vi "Mode 3 - GUI.vi"() -> ()   [LabVIEW 2020]
uses:
  <vilib>/Platform/TimedLoop/XDataNode/timing_clust.ctl
  <vilib>/Platform/TimedLoop/XDataNode/nitl_modes.ctl
  <vilib>/Platform/TimedLoop/XDataNode/wakeup.ctl
  <vilib>/Instr/_visa.llb/VISA Configure Serial Port (Instr).vi
  <vilib>/platform/TimedLoop/XDataNode/XDataNode.xnode
  <vilib>/Platform/TimedLoop/XDataNode/XDNodeRunTimeDep.lvlib
panel:
  in  "byte count":u32=31
  in  "Slider 3 Counter":i32
  out "Blue Workpiece":bool
  out "Counter Up ?":bool
  in  "Slider 2 Counter":i32
  in  "Slider 1 Counter":i32
  out "Green Workpiece":bool
  out "Red Workpiece":bool
  in  "STOP":bool
  in  "VISA resource name":refnum<visa-resource-name>
  out "Report Data":string
  # "TRAINER ARDUINO\nMPS SORTING STATION"
  # "Mechatronics Engineering 2nd Generation\n  Vocational High School 2 Bojonegoro\n2021"
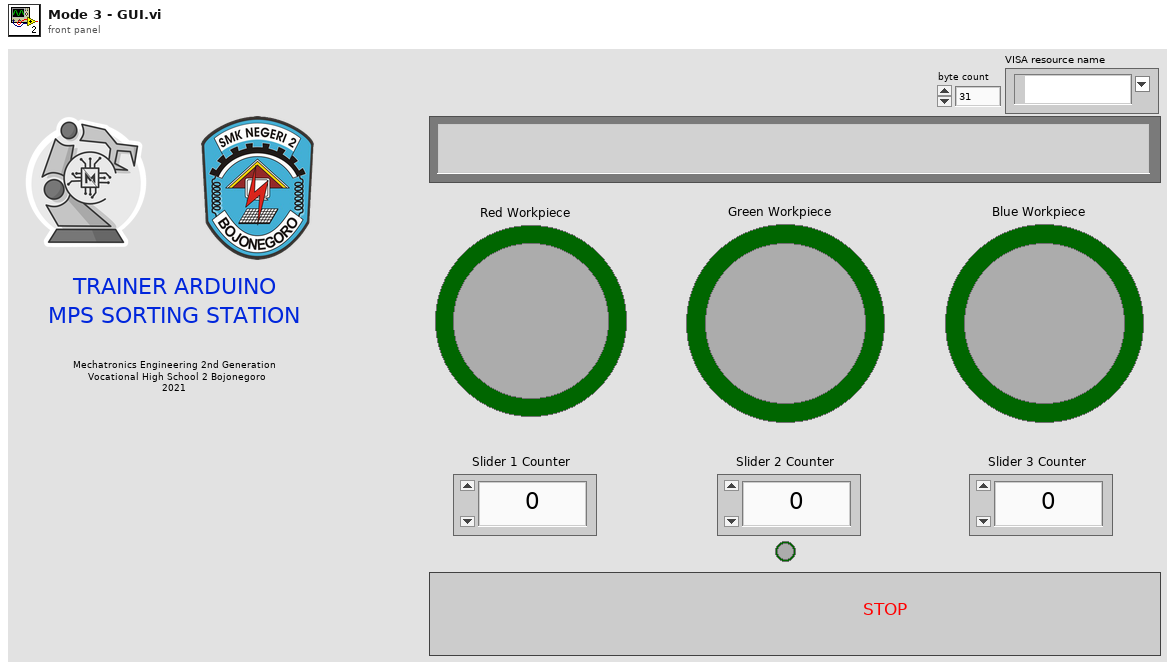
[diagram p1: front panel]
types:
  T1 = typedef "XDNodeRunTimeDep.lvlib/timing_clust.ctl" = cluster{"Expected End [f-1]":u64, "Actual End [f-1]":u64, "Finished Late? [f-1]":bool, "Expected End [i-1]":u64, "Actual End [i-1]":u64, "Finished Late? [i-1]":bool, "Expected Start [i]":u64, "Actual Start [i]":u64, "Expected Start [f]":u64, "Actual Start [f]":u64, "Source Name":string, "Structure Name":string, "Period":i64, "Deadline":i64, "Offset":i64, "Start":i64, "Priority":i32, "Timeout":i32, "Mode":T2, "Wakeup Reason":T3, "Error":errorcluster, "Source Type":string, "Secondary Source Type":string, "Global End Time":u64, "Global Start Time":u64, "Frame Duration":u64, "Iteration Duration":u64, "Assigned CPU":i32, "I/O Scan Engine Mode":u32}
  T2 = typedef "XDNodeRunTimeDep.lvlib/nitl_modes.ctl" = enum32{"No Change", "Process missed periods, maintain original phase", "Discard missed periods, maintain original phase", "Process missed periods, ignore original phase", "Discard missed periods, ignore original phase"}
  T3 = typedef "XDNodeRunTimeDep.lvlib/wakeup.ctl" = enum32{"Normal", "Aborted", "Asynchronous wakeup", "Timing source error", "Timed loop error", "Timeout"}
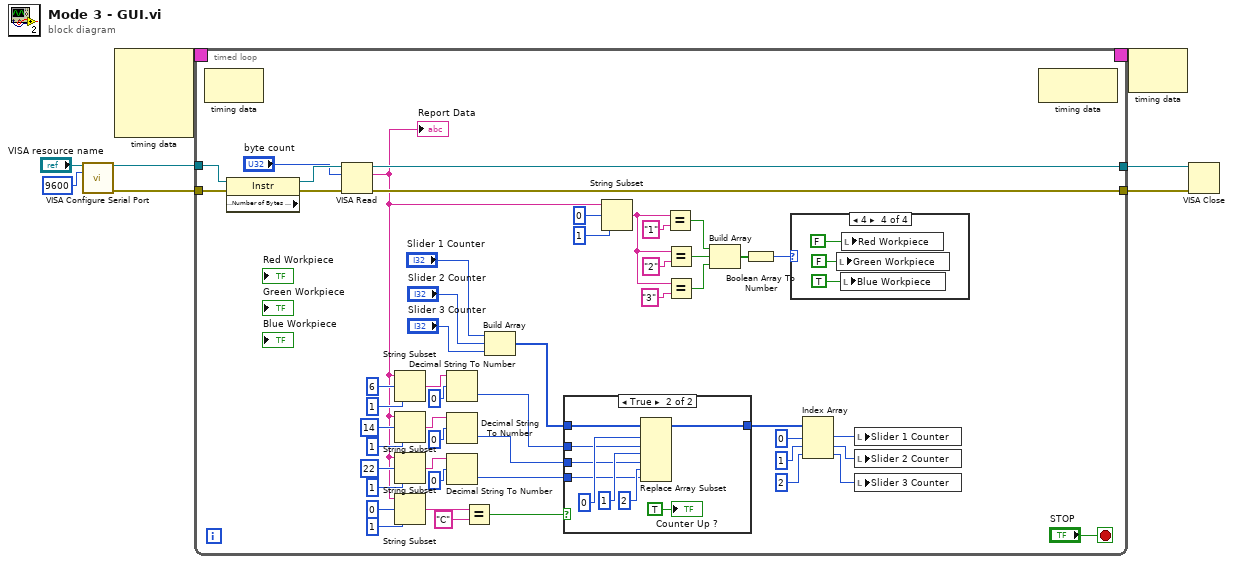
[diagram p0: block diagram]
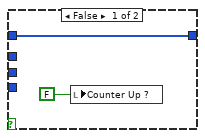
[diagram p2: hidden frame]
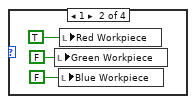
[diagram p4: hidden frame]
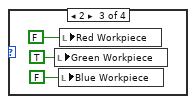
[diagram p5: hidden frame]
diagram:
  n1 = call-poly "VISA Configure Serial Port"("VISA resource name"="VISA resource name", "baud rate (9600)"=u32 9600) -> ("VISA resource name out"=w6:refnum<visa-resource-name>, "error out"=w5:errorcluster)  [unwired: 12 in]
  n2 = node-c288() -> (w8:T1)  [unwired: 4 in]
  n3 = timed-loop {
    timing: w8 -> [_]
    timing-out: [_] -> w7
    tunnel: w6 -> [w59]
    tunnel: w5 -> [w58]
    tunnel: [w55] -> w4
    tunnel: [w54] -> w3
    stop <- "STOP" stop-if-true
    n4 = node-c288() -> ()  [unwired: 1 in, 1 out]
    n5 = property class="Instr" props=["Serial Settings:Number of Bytes at Serial Port"](reference=w59, error in=w58) -> (reference out=w57:refnum<visa-resource-name>, error out=w56:errorcluster)  [unwired: 1 out]
    n6 = VISA Read(VISA resource name=w57, byte count="byte count", error in (no error)=w56) -> (VISA resource name out=w55:refnum<visa-resource-name>, read buffer=w20:string, error out=w54:errorcluster)  [unwired: 1 out]
    "Report Data" <- w20
    n7 = String Subset(string=w20, offset (0)=6, length (rest)=1 ("length (rest)")) -> (substring=w40:string)
    n8 = String Subset(string=w20, offset (0)=14, length (rest)=1 ("length (rest)")) -> (substring=w21:string)
    n9 = String Subset(string=w20, offset (0)=22, length (rest)=1 ("length (rest)")) -> (substring=w19:string)
    n10 = String Subset(string=w20, offset (0)=0, length (rest)=1 ("length (rest)")) -> (substring=w43:string)
    n11 = Decimal String To Number(string=w40, offset=0) -> (number=w37:i32)  [unwired: 1 in, 1 out]
    n12 = Decimal String To Number(string=w21, offset=0) -> (number=w36:i32)  [unwired: 1 in, 1 out]
    n13 = Decimal String To Number(string=w19, offset=0) -> (number=w16:i32)  [unwired: 1 in, 1 out]
    n14 = Equal?(x=w43, y="C") -> (x = y?=w41:bool)
    n15 = Build Array("Slider 1 Counter", "Slider 2 Counter", "Slider 3 Counter") -> (w35:i32[])
    n16 = case shown="True" w41 {
      tunnel: w37 -> [_ w68]
      tunnel: w36 -> [_ w67]
      tunnel: w35 -> [w61 w66]
      tunnel: [w61 w65] -> w34
      tunnel: w16 -> [_ w62]
      frame False {
        n17 = local write "Counter Up ?"(FALSE ("Boolean")) -> ()
      }
      frame True {
        n18 = Replace Array Subset(array=w66, new element #1=w68, index #1=0 ("index"), new element #2=w67, index #2=1 ("index"), new element #3=w62, index #3=2 ("index")) -> (w65:i32[])
        "Counter Up ?" <- TRUE ("Boolean")
      }
    }
    n19 = String Subset(string=w20, offset (0)=0, length (rest)=1 ("length (rest)")) -> (substring=w14:string)
    n20 = Equal?(x=w14, y="1") -> (x = y?=w11:bool)
    n21 = Equal?(x=w14, y="2") -> (x = y?=w12:bool)
    n22 = Equal?(x=w14, y="3") -> (x = y?=w13:bool)
    n23 = Build Array(w11, w12, w13) -> (w10:bool[])
    n24 = Boolean Array To Number(Boolean array=w10) -> (number=w9:u32)
    n25 = case shown="4" w9 {
      frame 0, Default {
      }
      frame 1 {
        n26 = local write "Green Workpiece"(FALSE ("Boolean")) -> ()
        n27 = local write "Blue Workpiece"(FALSE ("Boolean")) -> ()
        n28 = local write "Red Workpiece"(TRUE ("Boolean")) -> ()
      }
      frame 2 {
        n29 = local write "Green Workpiece"(TRUE ("Boolean")) -> ()
        n30 = local write "Blue Workpiece"(FALSE ("Boolean")) -> ()
        n31 = local write "Red Workpiece"(FALSE ("Boolean")) -> ()
      }
      frame 4 {
        n32 = local write "Green Workpiece"(FALSE ("Boolean")) -> ()
        n33 = local write "Blue Workpiece"(TRUE ("Boolean")) -> ()
        n34 = local write "Red Workpiece"(FALSE ("Boolean")) -> ()
      }
    }
    n35 = Index Array(array=w34, index #1=0 ("index"), index #2=1 ("index"), index #3=2 ("index")) -> (element #1=w30:i32, element #2=w31:i32, element #3=w17:i32)
    n36 = local write "Slider 1 Counter"(w30) -> ()
    n37 = local write "Slider 2 Counter"(w31) -> ()
    n38 = local write "Slider 3 Counter"(w17) -> ()
    n39 = node-c288() -> ()  [unwired: 1 in, 1 out]
  }
  n40 = node-c288(w7) -> ()  [unwired: 1 out]
  n41 = VISA Close(VISA resource name=w4, error in (no error)=w3) -> ()  [unwired: 1 out]
